vi "GetConditions.vi"(6 "condition type":T3, 7 "dg_op":string, 8 "error in (no error)":errorcluster, 11 "operating states in":variant) -> (0 "error out":errorcluster, 1 "expression":string, 2 "conditions":T1[](array[typedef]), 3 "operating states out":variant)   [LabVIEW 2017, in "Trigger.lvlib"]
uses:
  <vilib>/addons/InsightCM/Devices/Shared/Common/Trigger/Trigger.lvlib
  <vilib>/addons/InsightCM/Devices/Shared/Common/Trigger/controls/ConditionType.ctl
  <vilib>/addons/InsightCM/Devices/Shared/Common/Trigger/controls/TriggerCondition.ctl
  <vilib>/addons/InsightCM/MessageBus/Base/controls/Condition.ctl
  <vilib>/addons/InsightCM/Devices/Shared/Common/Trigger/controls/TriggerOperatingState.ctl
  <vilib>/addons/InsightCM/MessageBus/Base/controls/KeyValuePair.ctl
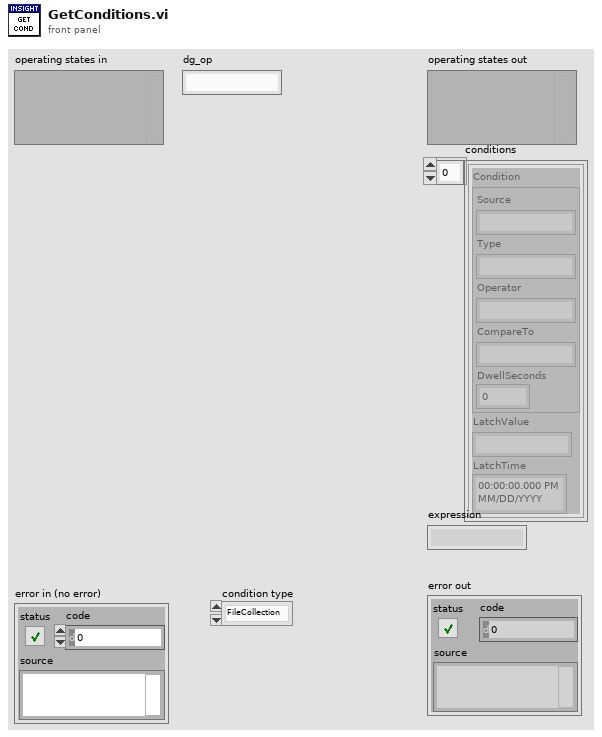
[diagram p1: front panel]
types:
  T1 = typedef "Trigger.lvlib/TriggerCondition.ctl" = cluster{"Condition":T2, "LatchValue":string, "LatchTime":timestamp}
  T2 = typedef "Condition.ctl" = cluster{"Source":string, "Type":string, "Operator":string, "CompareTo":string, "DwellSeconds":dbl}
  T3 = typedef "Trigger.lvlib/ConditionType.ctl" = enum16{"FileCollection", "TrendCollection"}
  T4 = typedef "Trigger.lvlib/TriggerOperatingState.ctl" = cluster{"Id":string, "Name":string, "Properties":T5[], "TrendExpression":string, "TrendConditions":T1[], "FileExpression":string, "FileConditions":T1[]}
  T5 = typedef "KeyValuePair.ctl" = cluster{"Key":string, "Value":string}
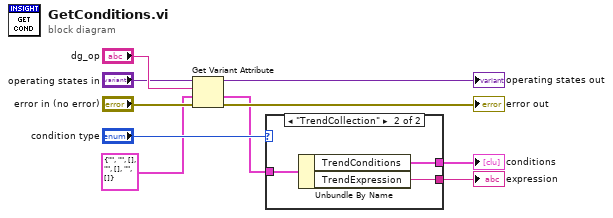
[diagram p0: block diagram]
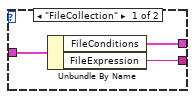
[diagram p2: hidden frame]
diagram:
  n1 = Get Variant Attribute(Variant="operating states in", name="dg_op", default value (empty Variant)=T4 {"Id"="", "Name"="", "Properties"=[], "TrendExpression"="", "TrendConditions"=[], "FileExpression"="", "FileConditions"=[]} ("OperatingState"), error in="error in (no error)") -> (duplicate Variant=→"operating states out":variant, value=w1:T4, error out=→"error out":errorcluster)  [unwired: 1 out]
  n2 = case shown="\"TrendCollection\"" "condition type" {
    tunnel: w1 -> [w13 w16]
    tunnel: [w12 w15] -> w5
    tunnel: [w11 w14] -> w4
    frame "FileCollection" {
      n3 = Unbundle By Name(w13) -> ("FileConditions"=w12:T1[], "FileExpression"=w11:string)
    }
    frame "TrendCollection" {
      n4 = Unbundle By Name(w16) -> ("TrendConditions"=w15:T1[], "TrendExpression"=w14:string)
    }
  }
  "conditions" <- w5
  "expression" <- w4
